vi "wait_&ackChar.vi"(8 "error in (no error)":errorcluster, 10 "caracter":string="1", 11 "VISA Refnum in":refnum<visa-resource-name>) -> (0 "error out":errorcluster, 3 "caracter leido":string)   [LabVIEW 2019]
uses:
  <vilib>/Utility/error.llb/Error Cluster From Error Code.vi
  <vilib>/ErrorRing/Error Ring.xnode
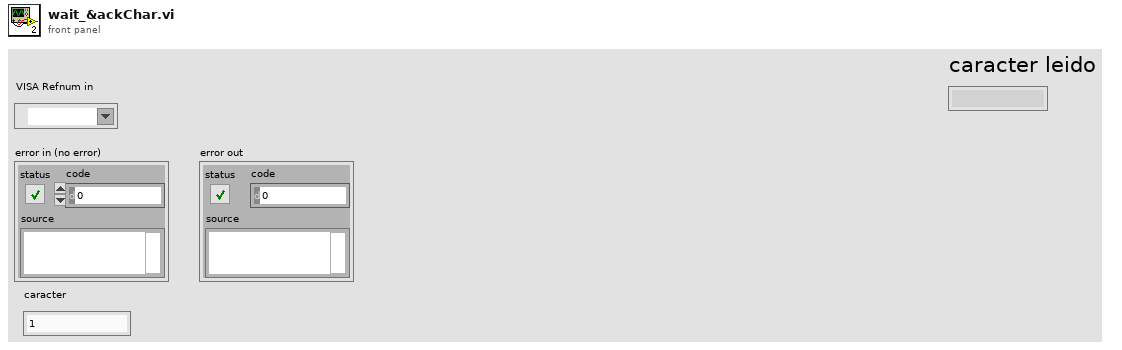
[diagram p1: front panel]
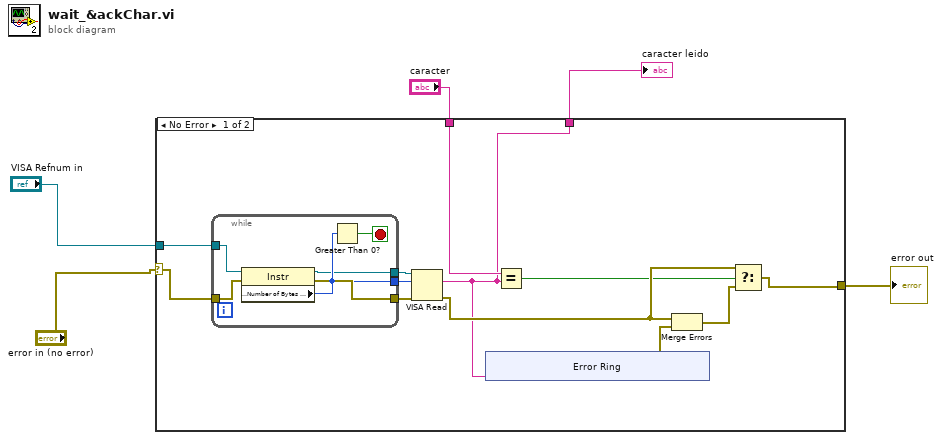
[diagram p0: block diagram]
diagram:
  n1 = case shown="No Error" "error in (no error)" {
    selector: "error in (no error)" -> [w8 w31]
    tunnel: "VISA Refnum in" -> [w16 _]
    tunnel: [w9 w31] -> w4
    tunnel: "caracter" -> [w7 _]
    tunnel: [w6 _] -> w1
    frame No Error {
      n2 = while {
        tunnel: w16 -> [w30]
        tunnel: [w28] -> w15
        tunnel: [w27] -> w17
        tunnel: [w26] -> w14
        tunnel: w8 -> [w25]
        stop <- w29 stop-if-true
        n3 = property class="Instr"(reference=w30, error in=w25) -> (reference out=w26:refnum<visa-resource-name>, error out=w28:errorcluster, "Serial Settings:Number of Bytes at Serial Port"=w27:u32)
        n4 = Greater Than 0?(x=w27) -> (x > 0?=w29:bool)
      }
      n5 = VISA Read(VISA resource name=w14, byte count=w17, error in (no error)=w15) -> (read buffer=w6:string, error out=w11:errorcluster)  [unwired: 2 out]
      n6 = xnode "Error Ring"("parameter 0"=w6) -> ("error out"=w13:errorcluster)
      n7 = Equal?(x=w7, y=w6) -> (x = y?=w10:bool)
      n8 = Merge Errors(w11, w13) -> (w12:errorcluster)
      n9 = Select(t=w11, s=w10, f=w12) -> (s? t:f=w9:errorcluster)
    }
    frame Error {
    }
  }
  "error out" <- w4
  "caracter leido" <- w1
